vi "Test App Removed Process Context Removed.vi"(8 "error in (no error)":errorcluster, 11 "Rig Test in":refnum<class "Application Test.lvclass">) -> (0 "error out":errorcluster, 3 "Rig Test out":refnum<class "Application Test.lvclass">)   [LabVIEW 2020, in "Application Test.lvclass"]
uses:
  Application Test.lvclass
  C:/Program Files (x86)/National Instruments/LabVIEW 2020/vi.lib/Asteme/LUnit/Test Case.lvclass
  Framework/Process/Process.lvclass
  Framework/Process/Process.lvclass/Process.ctl
  Framework/Application/Application.lvclass/Application.ctl
  <vilib>/Asteme/LUnit/Test Case.lvclass/Test Case.ctl
  <vilib>/Asteme/LUnit/LUnit Assertion Result.lvclass/LUnit Assertion Result.ctl
  Framework/Application/Private/Add Process to Map.vi
  Framework/Application/Private/Start Idle Processes if Running.vi
  Framework/Process/Protected/Messaging/Enqueue Message.vi
  Framework/Process/Public/Lifecycle/Get Lifecycle State.vi
  Framework/Process/Protected/SubVIs/Set Context.vi
  <vilib>/Asteme/LUnit/Palette/Pass.vi
  <vilib>/Asteme/LUnit/Palette/Fail.vi
  <vilib>/Asteme/LUnit/Variant to string.vi
  <vilib>/Asteme/LUnit/Set Assertion Type.vi
  Framework/Process/Private/SubVIs/Wait for finish.vi
  Framework/Process/Private/SubVIs/Set Lifecycle State.vi
  <vilib>/Utility/error.llb/Clear Errors.vi
  Framework/Process/Public/Lifecycle/Leave Process Loop.vi
  <vilib>/Asteme/LUnit/Add test result.vi
  <vilib>/Asteme/LUnit/LUnit Write Passed.vi
  <vilib>/Asteme/LUnit/LUnit Get Test Case.vi
  <vilib>/Asteme/LUnit/Assertion Result/LUnit Get Test Name.vi
  <vilib>/Asteme/LUnit/LUnit Write Message.vi
  <vilib>/Asteme/LUnit/LUnit Write Description.vi
  <vilib>/Asteme/LUnit/LUnit Write Assertion Type.vi
  <vilib>/Asteme/LUnit/Read Test Case Name.vi
  Framework/Application/Application.lvclass
  C:/Users/anton/Documents/GitHub/Triarc-Framework/source/Framework/Process/Process.lvclass
  <vilib>/Utility/error.llb/Error Cluster From Error Code.vi
  Framework/Application/Private/Throw Error If Process Already in App.vi
  Framework/Application/Private/Update Context for Owned Processes.vi
  <vilib>/Utility/Data Type/Get Type Information.vi
  <vilib>/Utility/LVClass/Get LV Class Name.vi
  <vilib>/Asteme/LUnit/LUnit Assertion Result.lvclass
  <vilib>/Asteme/LUnit/Test Case.lvclass
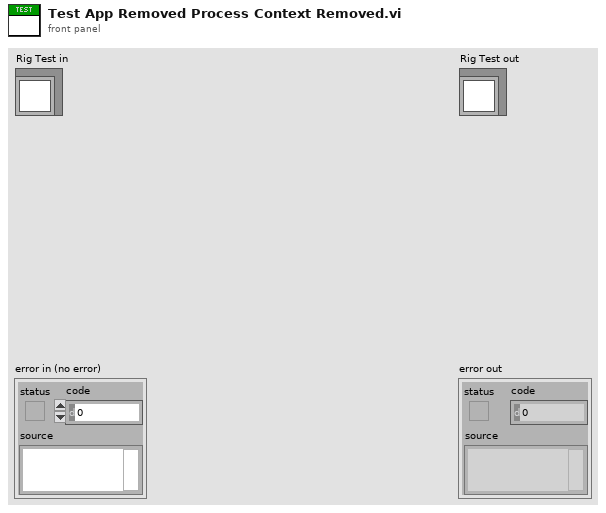
[diagram p1: front panel]
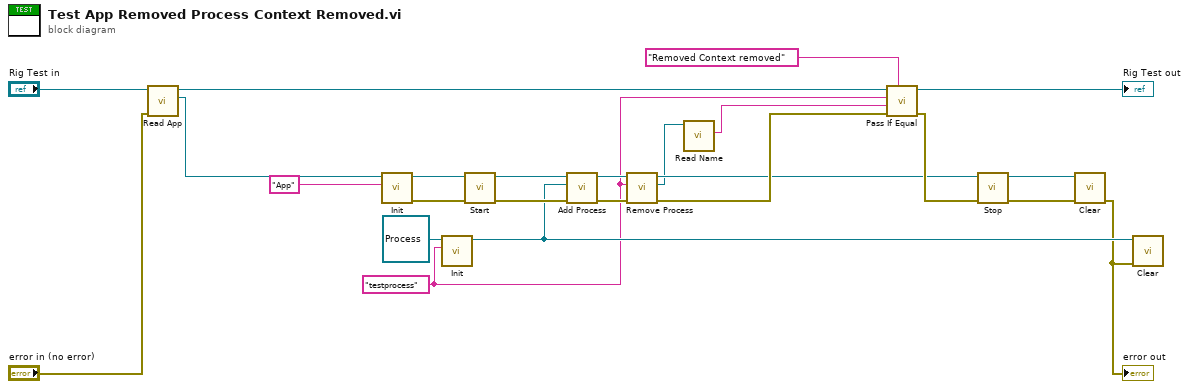
[diagram p0: block diagram]
diagram:
  w2 = "testprocess" ("Name")
  n1 = call "Read App.vi"("error in (no error)"="error in (no error)", "Application Test In"="Rig Test in") -> ("App out"=w23:refnum<class "Application.lvclass">, "Application Test Out"=w13:refnum<class "Application Test.lvclass">)  [unwired: 7 in, 1 out]
  n2 = call-dynamic "Init.vi"("Name"="App", "Process In"=w23) -> ("error out"=w14:errorcluster, "Process Out"=w15:refnum<class "Application.lvclass">)  [unwired: 8 in]
  n3 = call-dynamic "Init.vi"("Name"=w2, "Process In"=refnum<class "Process.lvclass"> refnum ("Process.lvclass")) -> ("Process Out"=w5:refnum<class "Process.lvclass">)  [unwired: 8 in, 1 out]
  n4 = call "Start.vi"("error in (no error)"=w14, "Process In"=w15) -> ("error out"=w16:errorcluster, "Process Out"=w6:refnum<class "Application.lvclass">)  [unwired: 7 in, 1 out]
  n5 = call "Add Process.vi"("error in (no error)"=w16, "Process"=w5, "Rig In"=w6) -> ("error out"=w20:errorcluster, "Rig Out"=w8:refnum<class "Application.lvclass">)  [unwired: 7 in]
  n6 = call "Remove Process.vi"("error in (no error)"=w20, "Process Name"=w2, "Rig In"=w8) -> ("error out"=w9:errorcluster, "App Process"=w3:refnum<class "Process.lvclass">, "Rig Out"=w7:refnum<class "Application.lvclass">)  [unwired: 6 in]
  n7 = call "Read Name.vi"("Process In"=w3) -> ("Qualified Name"=w1:string)  [unwired: 7 in, 3 out]
  n8 = call <vilib>:"Pass If Equal.vi"("Description"="Removed Context removed", "error in (no error)"=w9, "Actual"=w1, "Expected"=w2, "Test Case In"=w13) -> ("error out"=w18:errorcluster, "Test Case Out"=→"Rig Test out":refnum<class "Application Test.lvclass">)  [unwired: 5 in]
  n9 = call "Stop.vi"("error in (no error)"=w18, "Process In"=w7) -> ("error out"=w11:errorcluster, "Process Out"=w10:refnum<class "Application.lvclass">)  [unwired: 7 in, 1 out]
  n10 = call-dynamic "Clear.vi"("error in (no error)"=w11, "Application In"=w10) -> ("error out"=w4:errorcluster)  [unwired: 9 in]
  "error out" <- w4
  n11 = call-dynamic "Clear.vi"("error in (no error)"=w4, "Process In"=w5) -> ()  [unwired: 9 in, 1 out]
